vi "Get DG by DGNr.vi"(8 "error in (no error)":errorcluster, 10 "DG Nr.":i32=1 min=1, 11 "BME_DG_System in":refnum<class "BME_DG_System.lvclass">) -> (0 "error out":errorcluster, 1 "found?":bool, 2 "BME_DG_Base.lvclass":refnum<class "BME_DG_Base.lvclass">, 3 "BME_DG_System out":refnum<class "BME_DG_System.lvclass">)   [LabVIEW 2009, in "POLARIS BME DG.lvlib" / "BME_DG_System.lvclass"]
uses:
  BME_DG_System.lvclass
  BME_DG_Base/BME_DG_Base.lvclass
  BME_DG_System.lvclass/BME_DG_System.ctl
  POLARIS BME DG.lvlib
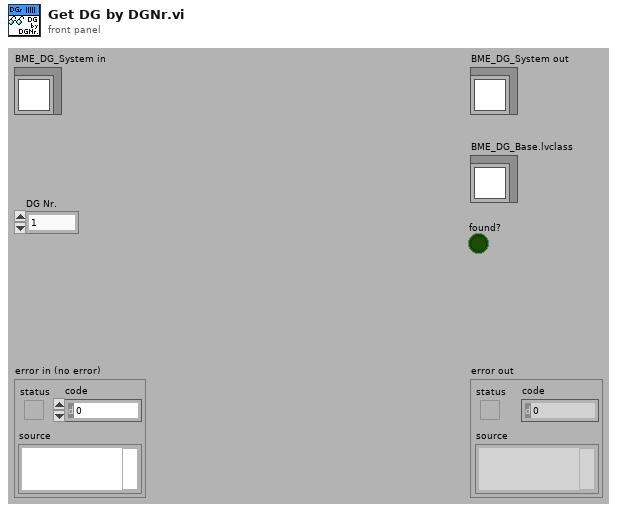
[diagram p1: front panel]
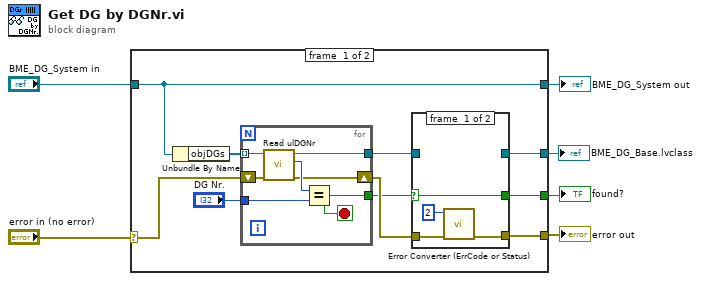
[diagram p0: block diagram]
diagram:
  n1 = case shown="No Error" "error in (no error)" {
    selector: "error in (no error)" -> [w12 w31]
    tunnel: [w11 w31] -> w5
    tunnel: [w16 w32] -> w3
    tunnel: "BME_DG_System in" -> [w16 w32]
    tunnel: [w10 _] -> w2
    tunnel: [w7 _] -> w1
    frame #0 {
      n2 = Unbundle By Name(w16) -> ("objDGs"=w15:refnum<class "BME_DG_Base.lvclass">[])
      n3 = for {
        tunnel: w15 -> [w30] mode=indexing
        tunnel: "DG Nr." -> [w28]
        tunnel: [w27] -> w9
        tunnel: [w26] -> w8
        shift-right: [w24] -> w13
        shift-left: w12 -> [w25]
        stop <- w26 stop-if-true
        n4 = call-dynamic "Read ulDGNr.vi"("error in (no error)"=w25, "BME_DG_Base in"=w30) -> ("error out"=w24:errorcluster, "ulDGNr"=w29:u32, "BME_DG_Base out"=w27:refnum<class "BME_DG_Base.lvclass">)  [unwired: 6 in, 1 out]
        n5 = Equal?(x=w29, y=w28) -> (x = y?=w26:bool)
      }
      n6 = case shown="False" w8 {
        selector: w8 -> [w17 w21]
        tunnel: w13 -> [w19 w22]
        tunnel: [w18 w22] -> w11
        tunnel: [_ w23] -> w10
        tunnel: w9 -> [_ w23]
        tunnel: [w17 w21] -> w7
        frame #0 {
          n7 = call "Error Converter (ErrCode or Status).vi"("error in (no error)"=w19, "error code"=2) -> ("error out"=w18:errorcluster)  [unwired: 9 in]
        }
        frame #1 {
        }
      }
    }
    frame #1 {
    }
  }
  "error out" <- w5
  "BME_DG_System out" <- w3
  "BME_DG_Base.lvclass" <- w2
  "found?" <- w1
